vi "Azimuth.vi"(0 "SP (pixels)":dbl=160.0, 5 "P-gain":dbl=1e-05, 7 "Deadband (pixels)":dbl=5.0, 11 "error in (no error)":errorcluster) -> (3 "Joystick Twist":dbl, 4 "PV (pixels)":dbl, 14 "Azimuth OK?":bool, 15 "error out":errorcluster)   [LabVIEW 2016]
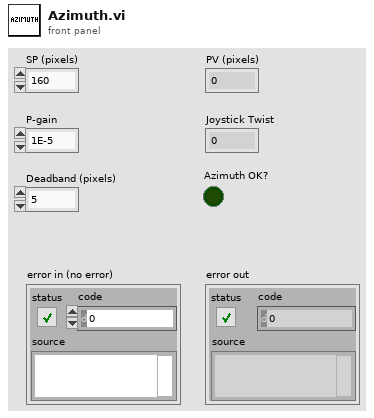
[diagram p1: front panel]
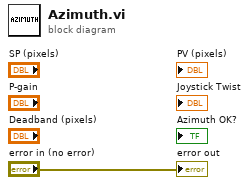
[diagram p0: block diagram]
diagram:
  "error out" <- "error in (no error)"
